vi "test Expedited Download U32 C5-E.vi"(11 "Test Case In":refnum<class "Tests SDO Manager.lvclass">) -> (0 "error out":errorcluster, 3 "Test Case Out":refnum<class "Tests SDO Manager.lvclass">)   [LabVIEW 2020, in "Tests SDO Manager.lvclass"]
uses:
  Tests SDO Manager.lvclass
  source/Logging/Logger/Logger.lvclass
  HAL/HAL-Devices/source/PCAN USB Dongle/PCAN Basic 4/Configure Strategies/Read-Write CAN Frame Strategy/PCAN Basic4 Read-Write CAN CC Frame Strategy.lvclass
  HAL/Source/Communicator/Communicator.lvclass
  <vilib>/ActorFramework/Stop Msg/Stop Msg.lvclass
  HAL/Source/Interfaces/IMessage/IMessage.lvclass
  Tests SDO Manager.lvclass/Tests SDO Manager.ctl
  source/SDO Manager/SDO Manager/SDO Manager/SDO Manager.lvclass
  <vilib>/ActorFramework/Actor/Actor.lvclass
  source/SDO Manager/SDO Manager/SDO Manager/Download U32.vi
  source/Typedefs/Multiplexer.ctl
  source/CANopen.lvlib
  <vilib>/Astemes/LUnit/Test Case.lvclass
  source/Logging/Log Level.vi
  source/Logging/CANopen Logging.lvlib
  source/SDO Manager/SDO Manager/SDO Transfer/SDO abort code.ctl
  source/SDO Manager/SDO Manager/SDO Transfer/SDO Transfer.lvclass
  source/Typedefs/SDO Result.ctl
panel:
  out "SDO Result":T1={"Success"=FALSE, "SDO abort code"={"Null"=TRUE, "Value"=84082688}, "Data"={"Null"=TRUE, "Data"=[]}} {"SDO abort code"."Value" items=["Toggle bit not allowed"=84082688, "SDO protocol timed out"=84148224, "Client/server command specifier not valid or unknown"=84148225, "Invalid block size (block mode only)"=84148226, "Invalid sequence number (block mode only)"=84148227, "CRC error (block mode only)"=84148228, "Out of memory"=84148229, "Attempt to read a write only object"=100728833, "Attempt to write a read only object"=100728834, "Object does not exist in the object dictionary"=100794368, "Object cannot be mapped to the PDO"=100925505, "The number and length of the objects to be mapped would exceed PDO length"=100925506, "General parameter incompatibility reason"=100925507, "General internal incompatibility in the device"=100925511, "Access failed due to an hardware error"=101056512, "Data type does not match, length of service parameter does not match"=101122064, "Data type does not match, length of service parameter too high"=101122066, "Data type does not match, length of service parameter too low"=101122067, "Sub-index does not exist"=101253137, "Invalid value for parameter (download only)"=101253168, "Value of parameter written too high (download only)"=101253169, "Value of parameter written too low (download only)"=101253170, "Maximum value is less than minimum value"=101253174, "Resource not available: SDO connection"=101318691, "General error"=134217728, "Data cannot be transferred or stored to the application"=134217760, "Data cannot be transferred or stored to the application because of local control"=134217761, "Data cannot be transferred or stored to the application because of the present device stable"=134217762, "Object dictionary dynamic generation fails or no object dictionary is present (e.g. object dictionary is generated from file and generation fails because of an file error)"=134217763, "No data available"=134217764]; "Data"."Data" format="%02x"}
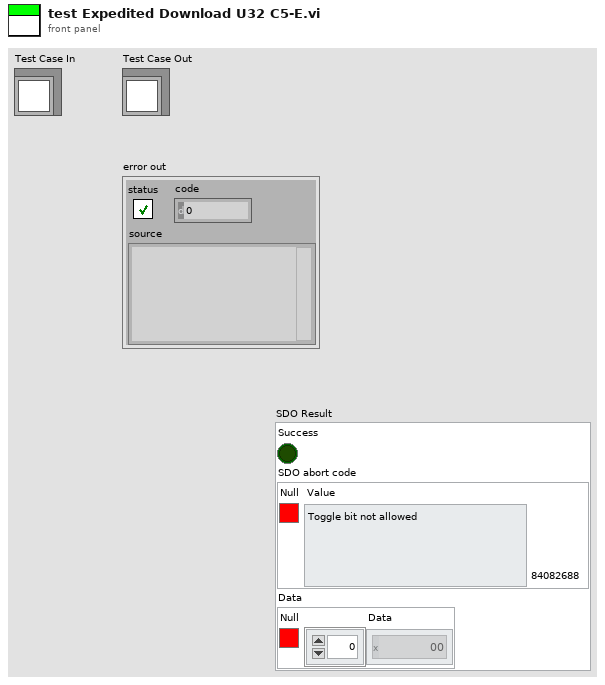
[diagram p1: front panel]
types:
  T1 = typedef "CANopen.lvlib/SDO Manager.lvlib/SDO Transfer.lvclass/SDO Result.ctl" = cluster{"Success":bool, "SDO abort code":cluster{"Null":bool, "Value":T2}, "Data":cluster{"Null":bool, "Data":u8[]}}
  T2 = typedef "CANopen.lvlib/SDO Manager.lvlib/SDO Transfer.lvclass/SDO abort code.ctl" = u32
  T3 = typedef "CANopen.lvlib/Multiplexer.ctl" = cluster{"Index":u16, "Sub Index":u8}
  T4 = enum16{"Error", "Warn", "Info", "Debug", "Trace"}
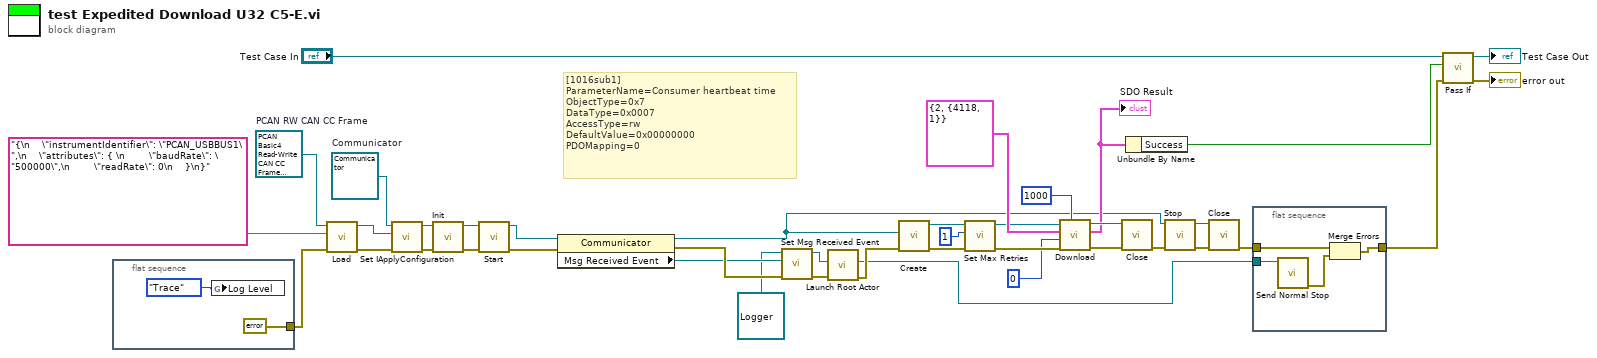
[diagram p0: block diagram]
diagram:
  w8 = refnum<class "Communicator.lvclass"> refnum  # Communicator
  w15 = refnum<class "PCAN Basic4 Read-Write CAN CC Frame Strategy.lvclass"> refnum  # PCAN RW CAN CC Frame
  # "[1016sub1]\nParameterName=Consumer heartbeat time\nObjectType=0x7\nDataType=0x0007\nAccessType=rw\nDefaultValue=0x00000000\nPDOMapping=0"
  n1 = flat-sequence {
    tunnel: [errorcluster {"status"=FALSE, "code"=0, "source"=""} ("error constant")] -> w13
    frame #0 {
      n2 = global write "Log Level.vi" "Log Level"(T4."Trace" ("Log Level")) -> ()
    }
  }
  n3 = call-dynamic "Load.vi"("error in"=w13, "Source"="{\n    \"instrumentIdentifier\": \"PCAN_USBBUS1\",\n    \"attributes\": { \n        \"baudRate\": \"500000\",\n        \"readRate\": 0\n    }\n}", "PCAN Basic Base Configure Strategy in"=w15) -> ("error out"=w11:errorcluster, "PCAN Basic Base Configure Strategy out"=w12:refnum<class "PCAN Basic4 Read-Write CAN CC Frame Strategy.lvclass">)  [unwired: 7 in]
  n4 = call-dynamic "Set IApplyConfiguration.vi"("Error In"=w11, "IApplyConfiguration"=w12, "Communicator in"=w8) -> ("Error Out"=w10:errorcluster, "Communicator out"=w9:refnum<class "Communicator.lvclass">)  [unwired: 7 in]
  n5 = call-dynamic "Init.vi"("Error In"=w10, "Communicator in"=w9) -> ("Error Out"=w7:errorcluster, "Communicator out"=w6:refnum<class "Communicator.lvclass">)  [unwired: 8 in]
  n6 = call-dynamic "Start.vi"("Error In"=w7, "Communicator in"=w6) -> ("Error Out"=w5:errorcluster, "Communicator out"=w4:refnum<class "Communicator.lvclass">)  [unwired: 8 in]
  n7 = property class="Communicator"(reference=w4, error in=w5) -> (reference out=w1:refnum<class "Communicator.lvclass">, error out=w30:errorcluster, "Msg Received Event"=w29:refnum<user-event>)
  n8 = call "Set Msg Received Event.vi"("error in"=w30, "Msg Received Event"=w29, "Logger in"=refnum<class "Logger.lvclass"> refnum) -> ("error out"=w32:errorcluster, "Logger out"=w31:refnum<class "Logger.lvclass">)  [unwired: 7 in]
  n9 = call <vilib>:"Launch Root Actor.vi"("error in (no error)"=w32, "Actor"=w31) -> ("error out"=w28:errorcluster, "Actor's Enqueuer"=w25:refnum<class "Message Enqueuer.lvclass">)  [unwired: 8 in]
  n10 = call "Create.vi"("Error In"=w28, "ICommunicate"=w1) -> ("Error Out"=w23:errorcluster, "SDO Manager"=w22:refnum<class "SDO Manager.lvclass">)  [unwired: 8 in]
  n11 = call "Set Max Retries.vi"("error in"=w23, "Max Retries"=u8 1, "SDO Manager in"=w22) -> ("error out"=w20:errorcluster, "SDO Manager out"=w21:refnum<class "SDO Manager.lvclass">)  [unwired: 7 in]
  n12 = call-poly "Download.vi"("Timeout"=1000, "error in"=w20, "Value"=u32 0, "Parameters"=cluster{"Node-ID":u8, "Multiplexer":T3} {"Node-ID"=2, "Multiplexer"={"Index"=4118, "Sub Index"=1}}, "SDO Manager in"=w21) -> ("error out"=w35:errorcluster, "SDO Result"=w33:T1, "SDO Manager out"=w34:refnum<class "SDO Manager.lvclass">)  [unwired: 4 in]
  "SDO Result" <- w33
  n13 = call "Close.vi"("Error In"=w35, "SDO Manager"=w34) -> ("Error Out"=w37:errorcluster)  [unwired: 8 in, 1 out]
  n14 = Unbundle By Name(w33) -> ("Success"=w18:bool)
  n15 = call-dynamic "Stop.vi"("Error In"=w37, "Communicator in"=w1) -> ("Error Out"=w3:errorcluster, "Communicator out"=w2:refnum<class "Communicator.lvclass">)  [unwired: 8 in]
  n16 = call-dynamic "Close.vi"("Error In"=w3, "Communicator in"=w2) -> ("Error Out"=w26:errorcluster)  [unwired: 8 in, 1 out]
  n17 = flat-sequence {
    tunnel: w26 -> [w43]
    tunnel: w25 -> [w46]
    tunnel: [w44] -> w24
    frame #0 {
      n18 = call <vilib>:"Send Normal Stop.vi"("Message Enqueuer"=w46) -> ("error out"=w45:errorcluster)  [unwired: 10 in]
      n19 = Merge Errors(w43, w45) -> (w44:errorcluster)
    }
  }
  n20 = call <vilib>:"Pass If.vi"("error in (no error)"=w24, "Pass?"=w18, "LUnit Test Case In"="Test Case In") -> ("error out"=→"error out":errorcluster, "LUnit Test Case Out"=→"Test Case Out":refnum<class "Tests SDO Manager.lvclass">)  [unwired: 7 in]
